vi "Servo Control.vi"() -> ()   [LabVIEW 2025]
panel:
  in  "Angulo":u8(slide) scale=0.0..180.0
  out "read buffer":string
  in  "stop":bool
  out "error out":errorcluster
  in  "Pin":u8=4 min=4 max=40
  in  "VISA resource name":refnum<visa-resource-name>
  # "Ejemplo: Control de Servo\nEste ejemplo muestra cómo controlar la posición de un servomotor en LV_ESP32, permitiendo asignar un ángulo de rotación entre 0° y 180° y actualizar su posición en tiempo real.\n\nEntradas requeridas:\n\nPin_Servo: Pin al que está conectado el servo.\n\nÁngulo: Valor de rotación deseado para el servo (0° a 180°).\n\nSalidas generadas:\n\nPosición física del servo según el ángulo asignado."
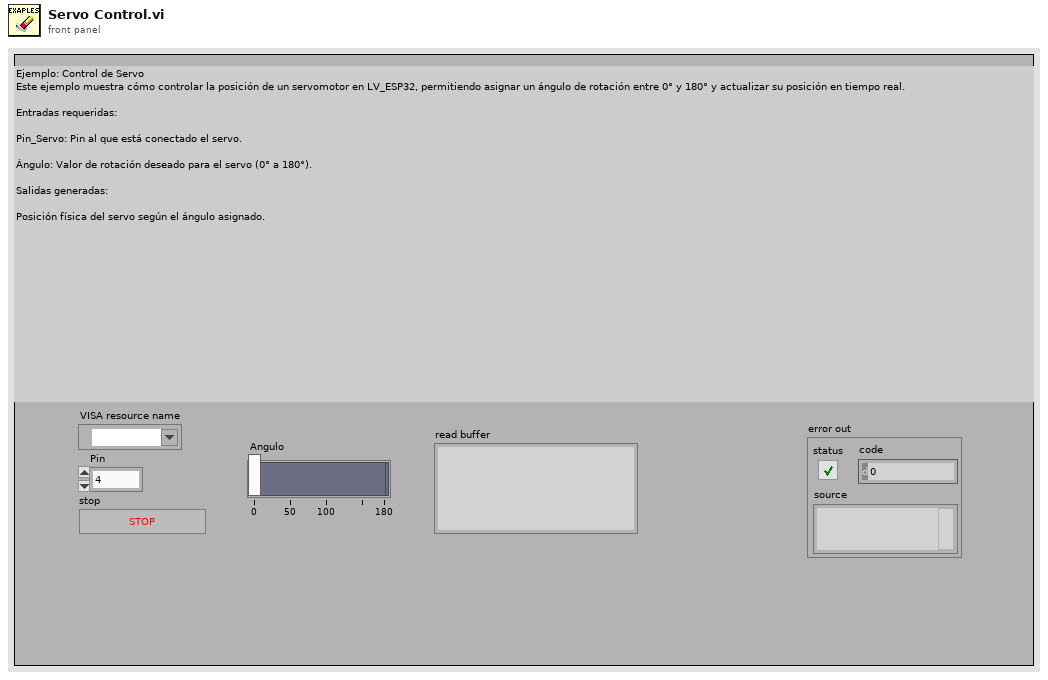
[diagram p1: front panel]
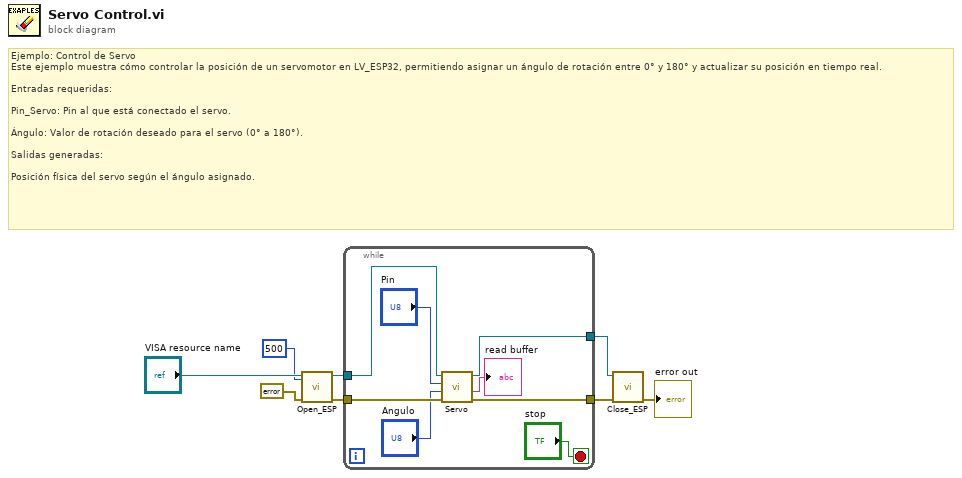
[diagram p0: block diagram]
diagram:
  # "Ejemplo: Control de Servo\nEste ejemplo muestra cómo controlar la posición de un servomotor en LV_ESP32, permitiendo asignar un ángulo de rotación entre 0° y 180° y actualizar su posición en tiempo real.\n\nEntradas requeridas:\n\nPin_Servo: Pin al que está conectado el servo.\n\nÁngulo: Valor de rotación deseado para el servo (0° a 180°).\n\nSalidas generadas:\n\nPosición física del servo según el ángulo asignado."
  n1 = call "Open_ESP.vi"("timeout (10sec)"=u32 500, "error in (no error)"=errorcluster {"status"=FALSE, "code"=0, "source"=""}, "VISA resource name"="VISA resource name") -> ("error out"=w4:errorcluster, "VISA resource name out"=w5:refnum<visa-resource-name>)  [unwired: 7 in]
  n2 = while {
    tunnel: w5 -> [w16]
    tunnel: w4 -> [w15]
    tunnel: [w14] -> w3
    tunnel: [w13] -> w2
    stop <- "stop" stop-if-true
    n3 = call "Servo.vi"("error in (no error)"=w15, "Angulo"="Angulo", "Pin"="Pin", "VISA resource name"=w16) -> ("error out"=w14:errorcluster, "read buffer"=→"read buffer":string, "VISA resource name out"=w13:refnum<visa-resource-name>)  [unwired: 5 in]
  }
  n4 = call "Close_ESP.vi"("error in (no error)"=w3, "VISA resource name"=w2) -> ("error out"=→"error out":errorcluster)  [unwired: 9 in]
